vi "Check Subscription Policy.vi"(8 "error in (no error)":errorcluster, 11 "Subscription Policy":T1) -> (0 "error out (Unsubscribe?)":errorcluster, 3 "Subscription Policy Out":T1)   [LabVIEW 2018, in "MVA Framework.lvlib" / "IMediator.lvlib" / "ISubscriptionPolicy.lvclass"]
doc: "检查订阅政策"
uses:
  ISubscriptionPolicy.lvclass
  ISubscriptionPolicy Reference.ctl
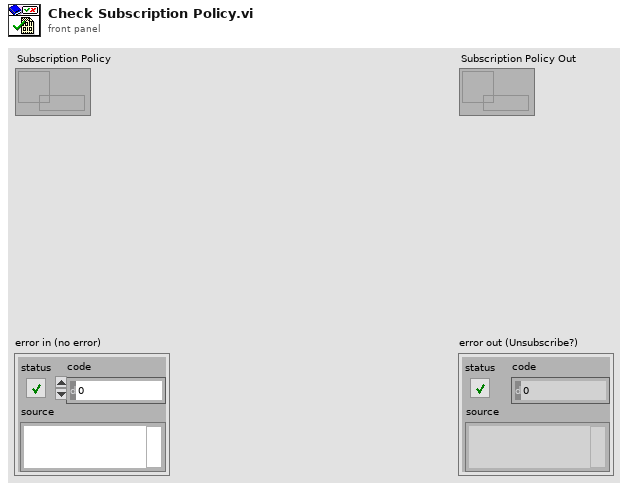
[diagram p1: front panel]
types:
  T1 = typedef "MVA Framework.lvlib/IMediator.lvlib/ISubscriptionPolicy.lvclass/ISubscriptionPolicy Reference.ctl" = refnum<data-value>
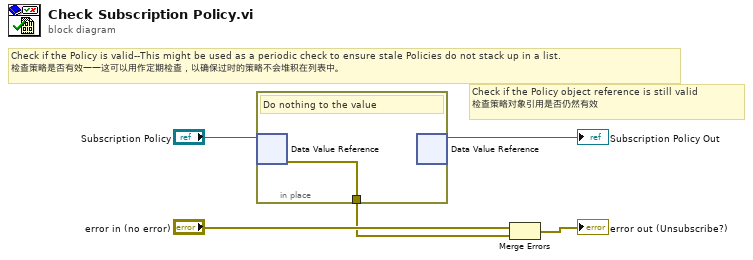
[diagram p0: block diagram]
diagram:
  # "Check if the Policy object reference is still valid\n检查策略对象引用是否仍然有效"
  # "Check if the Policy is valid--This might be used as a periodic check to ensure stale Policies do not stack up in a list.\n检查策略是否有效——这可以用作定期检查，以确保过时的策略不会堆积在列表中。"
  n1 = in-place {
    in-place-border: [w6] -> w2
    # "Do nothing to the value"
    n2 = in-place-dvr #1("Subscription Policy") -> (w6:errorcluster)  [unwired: 1 out]
    n3 = in-place-dvr #1() -> (→"Subscription Policy Out":T1)  [unwired: 1 in, 1 out]
  }
  n4 = Merge Errors("error in (no error)", w2) -> (→"error out (Unsubscribe?)":errorcluster)
